vi "Aerotech Joystick Control Tester.vi"() -> ()   [LabVIEW 2017]
uses:
  Shared Components/Gantry Class/Type Definitions/Virtual Modes.ctl
  Shared Components/Config Manager Class/Type Definitions/Camera Enum.ctl
  Shared Components/Gantry Class/Type Definitions/Init_Modes.ctl
  Shared Components/WorkTable Class/Type Definitions/Worktable_Syringe.ctl
  Shared Components/Vec3d Class/Vec3d Class.lvclass
  Shared Components/Config Manager Class/Type Definitions/Potting Surface Type.ctl
  Shared Components/Gantry Class/Gantry Class.lvclass
  Shared Components/SyringeTool Class/SyringeTool Class.lvclass
  Shared Components/WorkTable Class/WorkTable Class.lvclass
panel:
  in  "Camera Name":T1
  in  "Virtual Mode":T2
  in  "HOME?":bool=TRUE
  in  "stop":bool
  out "Image":T3(plugin-control)
  out "error out":errorcluster
  in  "Config Folder":path=path "C:/Users/Admin/Gantry Purdue/pixel-gantry-control/Config"
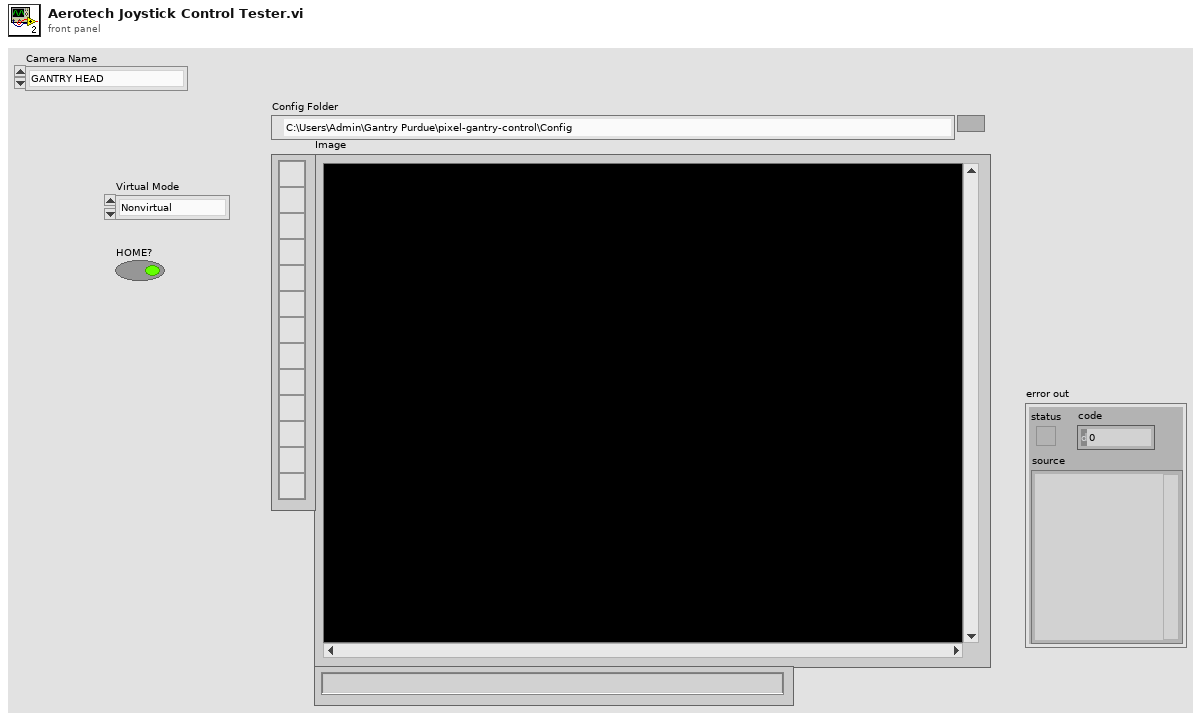
[diagram p1: front panel]
types:
  T1 = typedef "Camera Enum.ctl" = enum16{"GANTRY HEAD", "NEEDLE CALIBRATION X", "NEEDLE CALIBRATION Y", "STAND CAMERA"}
  T2 = typedef "Virtual Modes.ctl" = enum16{"Nonvirtual", "Pseudovirtual", "Virtual"}
  T3 = typedef "IMAQ Image.ctl" = refnum<image>
  T4 = typedef "Potting Surface Type.ctl" = enum16{"default", "hdi_edge_pads", "bbm_edge_pads", "address_pads"}
  T5 = typedef "Worktable_Syringe.ctl" = cluster{"Syringe Holder":enum16{"Empty", "Populated", "Calibrated"}, "Mixing Time":timestamp, "Tip Offset":refnum<class "Vec3d Class.lvclass">}
  T6 = typedef "Init_Modes.ctl" = enum16{"Full", "Robot Only", "Dispenser Only", "Cameras Only", "Robot and Cameras", "Robot and Cameras and Dispenser", "Manifold Only"}
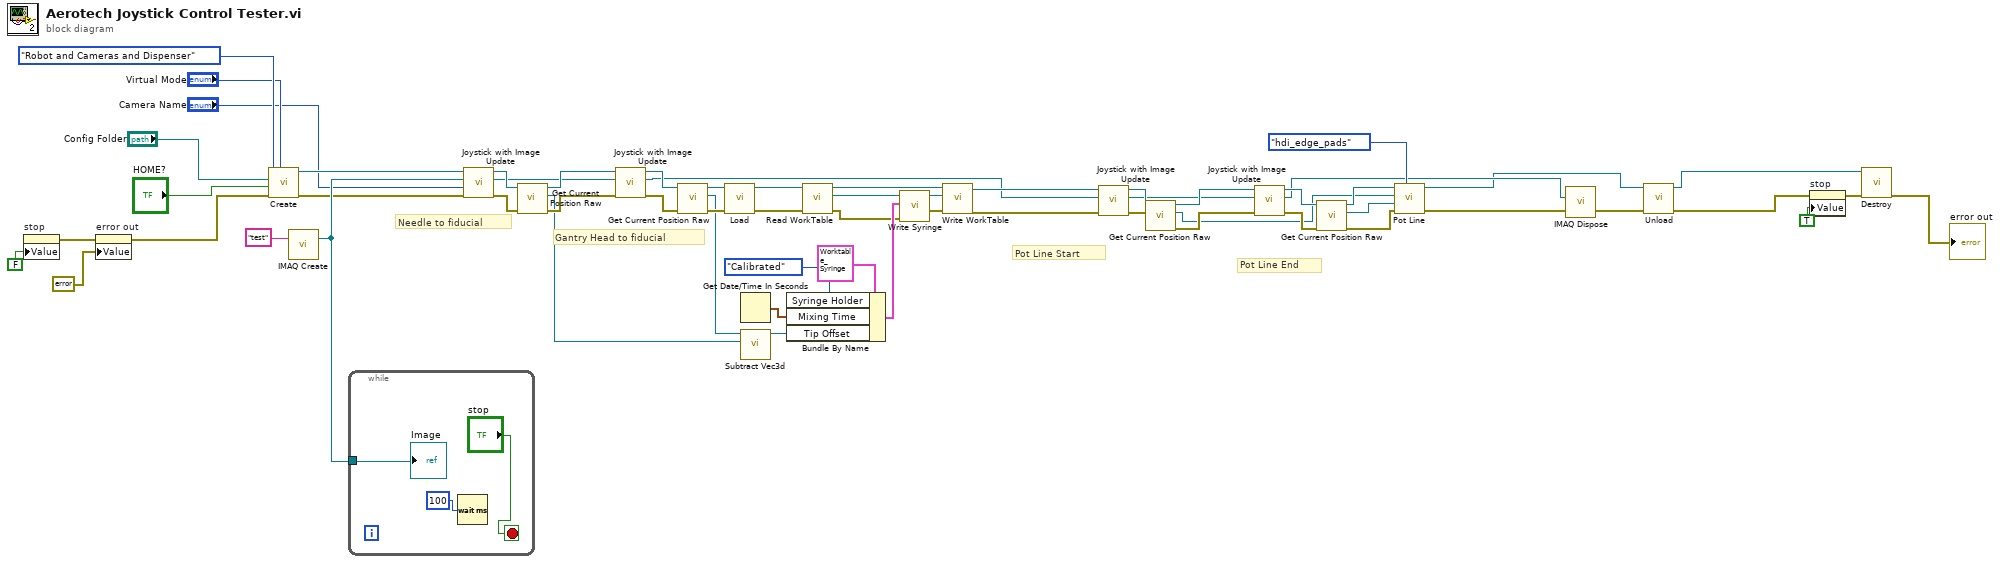
[diagram p0: block diagram]
diagram:
  # "Pot Line End"
  # "Gantry Head to fiducial"
  # "Pot Line Start"
  # "Needle to fiducial"
  n1 = property on="stop" class="Bool (strict)"("Value"=FALSE) -> (error out=w5:errorcluster)  [unwired: 2 in, 1 out]
  n2 = property on="error out" class="Clust (strict)"(error in=w5, "Value"=errorcluster {"status"=FALSE, "code"=0, "source"=""} ("error in (no error)")) -> (error out=w4:errorcluster)  [unwired: 1 in, 1 out]
  n3 = call "Create.vi"("Virtual Mode"="Virtual Mode", "error in"=w4, "HOME?"="HOME?", "Config Folder"="Config Folder", "Init Mode"=Init_Modes."Robot and Cameras and Dispenser") -> ("error out"=w53:errorcluster, "Gantry out"=w55:refnum<class "Gantry Class.lvclass">)  [unwired: 5 in]
  n4 = call "IMAQ Create"("Image Name"="test") -> ("New Image"=w54:T3)  [unwired: 4 in, 1 out]
  n5 = while {
    tunnel: w54 -> [w63]
    stop <- "stop" stop-if-true
    n6 = Wait (ms)(milliseconds to wait=u32 100) -> ()  [unwired: 1 out]
    "Image" <- w63
  }
  n7 = call-dynamic "Joystick with Image Update.vi"("error in (no error)"=w53, "Camera Name"="Camera Name", "Image In"=w54, "Gantry Class in"=w55) -> ("error out"=w48:errorcluster, "Image Out"=w46:T3, "Gantry Class out"=w49:refnum<class "Gantry Class.lvclass">)  [unwired: 5 in]
  n8 = call-dynamic "Get Current Position Raw.vi"("error in"=w48, "Gantry in"=w49) -> ("error out"=w45:errorcluster, "Vec3d Class out"=w6:refnum<class "Vec3d Class.lvclass">, "Gantry out"=w47:refnum<class "Gantry Class.lvclass">)  [unwired: 7 in]
  n9 = call-dynamic "Joystick with Image Update.vi"("error in (no error)"=w45, "Image In"=w46, "Gantry Class in"=w47) -> ("error out"=w43:errorcluster, "Image Out"=w19:T3, "Gantry Class out"=w44:refnum<class "Gantry Class.lvclass">)  [unwired: 6 in]
  n10 = call-dynamic "Get Current Position Raw.vi"("error in"=w43, "Gantry in"=w44) -> ("error out"=w41:errorcluster, "Vec3d Class out"=w7:refnum<class "Vec3d Class.lvclass">, "Gantry out"=w42:refnum<class "Gantry Class.lvclass">)  [unwired: 7 in]
  n11 = call "Load.vi"("error in"=w41, "Gantry in"=w42) -> ("error out"=w39:errorcluster, "SyringeTool out"=w40:refnum<class "SyringeTool Class.lvclass">)  [unwired: 8 in]
  n12 = Get Date/Time In Seconds() -> (seconds since 1Jan1904=w33:timestamp)
  n13 = call "Subtract Vec3d.vi"("Vec3d in 2"=w6, "Vec3d in 1"=w7) -> ("Vec3d Class out"=w34:refnum<class "Vec3d Class.lvclass">)  [unwired: 8 in, 1 out]
  n14 = Bundle By Name(cluster=T5 {"Syringe Holder"=enum."Empty", "Mixing Time"=timestamp(0 s since 1904-01-01), "Tip Offset"=refnum} ("Syringe"), "Syringe Holder"=enum16{"Empty", "Populated", "Calibrated"}."Calibrated", "Mixing Time"=w33, "Tip Offset"=w34) -> (w36:T5)
  n15 = call-dynamic "Read WorkTable.vi"("error in"=w39, "Gantry Class in"=w40) -> ("error out"=w30:errorcluster, "WorkTable Class.lvclass"=w38:refnum<class "WorkTable Class.lvclass">, "Gantry Class out"=w32:refnum<class "SyringeTool Class.lvclass">)  [unwired: 7 in]
  n16 = call-dynamic "Write Syringe.vi"("error in (no error)"=w30, "Syringe"=w36, "WorkTable Class in"=w38) -> ("error out"=w29:errorcluster, "WorkTable Class out"=w31:refnum<class "WorkTable Class.lvclass">)  [unwired: 7 in]
  n17 = call-dynamic "Write WorkTable.vi"("error in (no error)"=w29, "WorkTable Class.lvclass"=w31, "Gantry Class in"=w32) -> ("error out"=w20:errorcluster, "Gantry Class out"=w21:refnum<class "SyringeTool Class.lvclass">)  [unwired: 7 in]
  n18 = call-dynamic "Joystick with Image Update.vi"("error in (no error)"=w20, "Image In"=w19, "Gantry Class in"=w21) -> ("error out"=w27:errorcluster, "Image Out"=w25:T3, "Gantry Class out"=w28:refnum<class "SyringeTool Class.lvclass">)  [unwired: 6 in]
  n19 = call-dynamic "Get Current Position Raw.vi"("error in"=w27, "Gantry in"=w28) -> ("error out"=w24:errorcluster, "Vec3d Class out"=w17:refnum<class "Vec3d Class.lvclass">, "Gantry out"=w26:refnum<class "SyringeTool Class.lvclass">)  [unwired: 7 in]
  n20 = call-dynamic "Joystick with Image Update.vi"("error in (no error)"=w24, "Image In"=w25, "Gantry Class in"=w26) -> ("error out"=w22:errorcluster, "Image Out"=w12:T3, "Gantry Class out"=w23:refnum<class "SyringeTool Class.lvclass">)  [unwired: 6 in]
  n21 = call-dynamic "Get Current Position Raw.vi"("error in"=w22, "Gantry in"=w23) -> ("error out"=w15:errorcluster, "Vec3d Class out"=w16:refnum<class "Vec3d Class.lvclass">, "Gantry out"=w18:refnum<class "SyringeTool Class.lvclass">)  [unwired: 7 in]
  n22 = call-dynamic "Pot Line.vi"("Potting Surface Type"=Potting_Surface_Type."hdi_edge_pads", "error in"=w15, "End Position"=w16, "Start Position"=w17, "SyringeTool in"=w18) -> ("error out"=w13:errorcluster, "SyringeTool out"=w11:refnum<class "SyringeTool Class.lvclass">)  [unwired: 5 in]
  n23 = call "IMAQ Dispose"("Image"=w12, "error in (no error)"=w13) -> ("error out"=w10:errorcluster)  [unwired: 4 in]
  n24 = call "Unload.vi"("error in"=w10, "SyringeTool in"=w11) -> ("error out"=w9:errorcluster, "Gantry out"=w8:refnum<class "Gantry Class.lvclass">)  [unwired: 8 in]
  n25 = property on="stop" class="Bool (strict)"(error in=w9, "Value"=TRUE) -> (error out=w52:errorcluster)  [unwired: 1 in, 1 out]
  n26 = call "Destroy.vi"("error in"=w52, "Gantry Class in"=w8) -> ("error out"=→"error out":errorcluster)  [unwired: 9 in]
